vi "P3-3.vi"() -> ()   [LabVIEW 2011]
panel:
  out "위험!":bool
  out "킬로그램":dbl
  in  "파운드":dbl
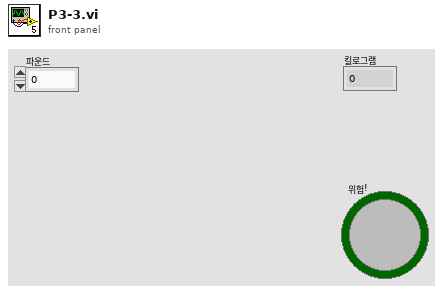
[diagram p1: front panel]
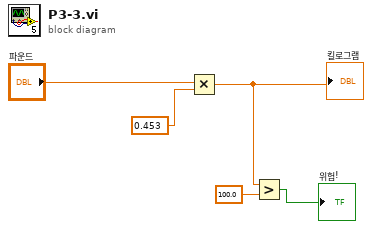
[diagram p0: block diagram]
diagram:
  n1 = Multiply(x="파운드", y=0.453) -> (x*y=w3:dbl)
  "킬로그램" <- w3
  n2 = Greater?(x=w3, y=100.0) -> (0:→"위험!":bool)
